vi "平均取樣數值適應性控制.vi"() -> ()   [LabVIEW 2010]
panel:
  in  "number of samples":i32=100
  in  "rate":dbl=1000.0
  in  "連續取樣多少誤差個數符合條件時算收斂":dbl=10.0
  in  "負誤差範圍%":dbl=-10.0
  in  "正誤差範圍%":dbl=10.0
  out "理想系統與FIR輸出":cluster{dbl, dbl}(graph)
  out "收斂時間":dbl
  out "Boolean":bool
  out "當下符合誤差條件數":dbl
  out "每次迴圈運時時間(ms)":u32
  out "當下誤差%":dbl
  out "error out":errorcluster
  out "system輸出":dbl
  out "input_x(t)":dbl(graph)
  out "ERR":dbl(graph)
  out "權重函數向量":dbl[](array[numeric])
  in  "order":i32=8
  out "LMS":dbl[](graph)
  out "FIR輸出":dbl
  in  "Stop Button":bool
  in  "u(收斂係數)":dbl=0.005
  # "A0:模擬輸入 pulse_output 2"
  # "A1:理想系統 pulse_output 1"
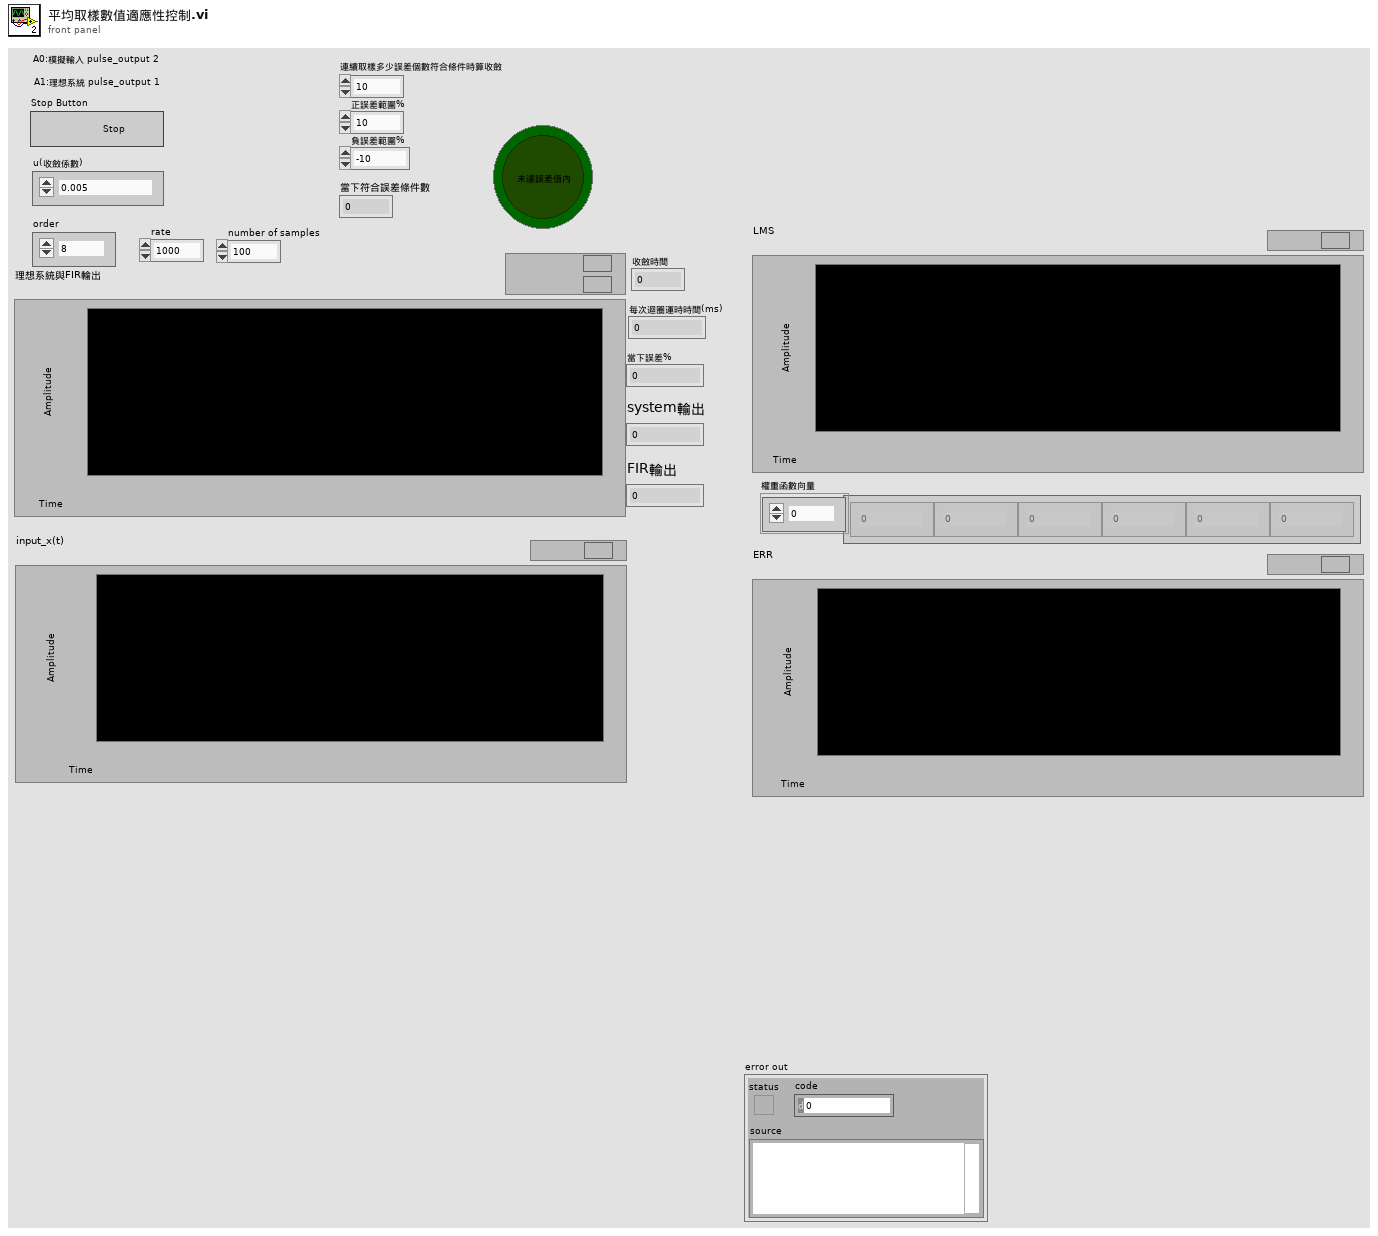
[diagram p1: front panel]
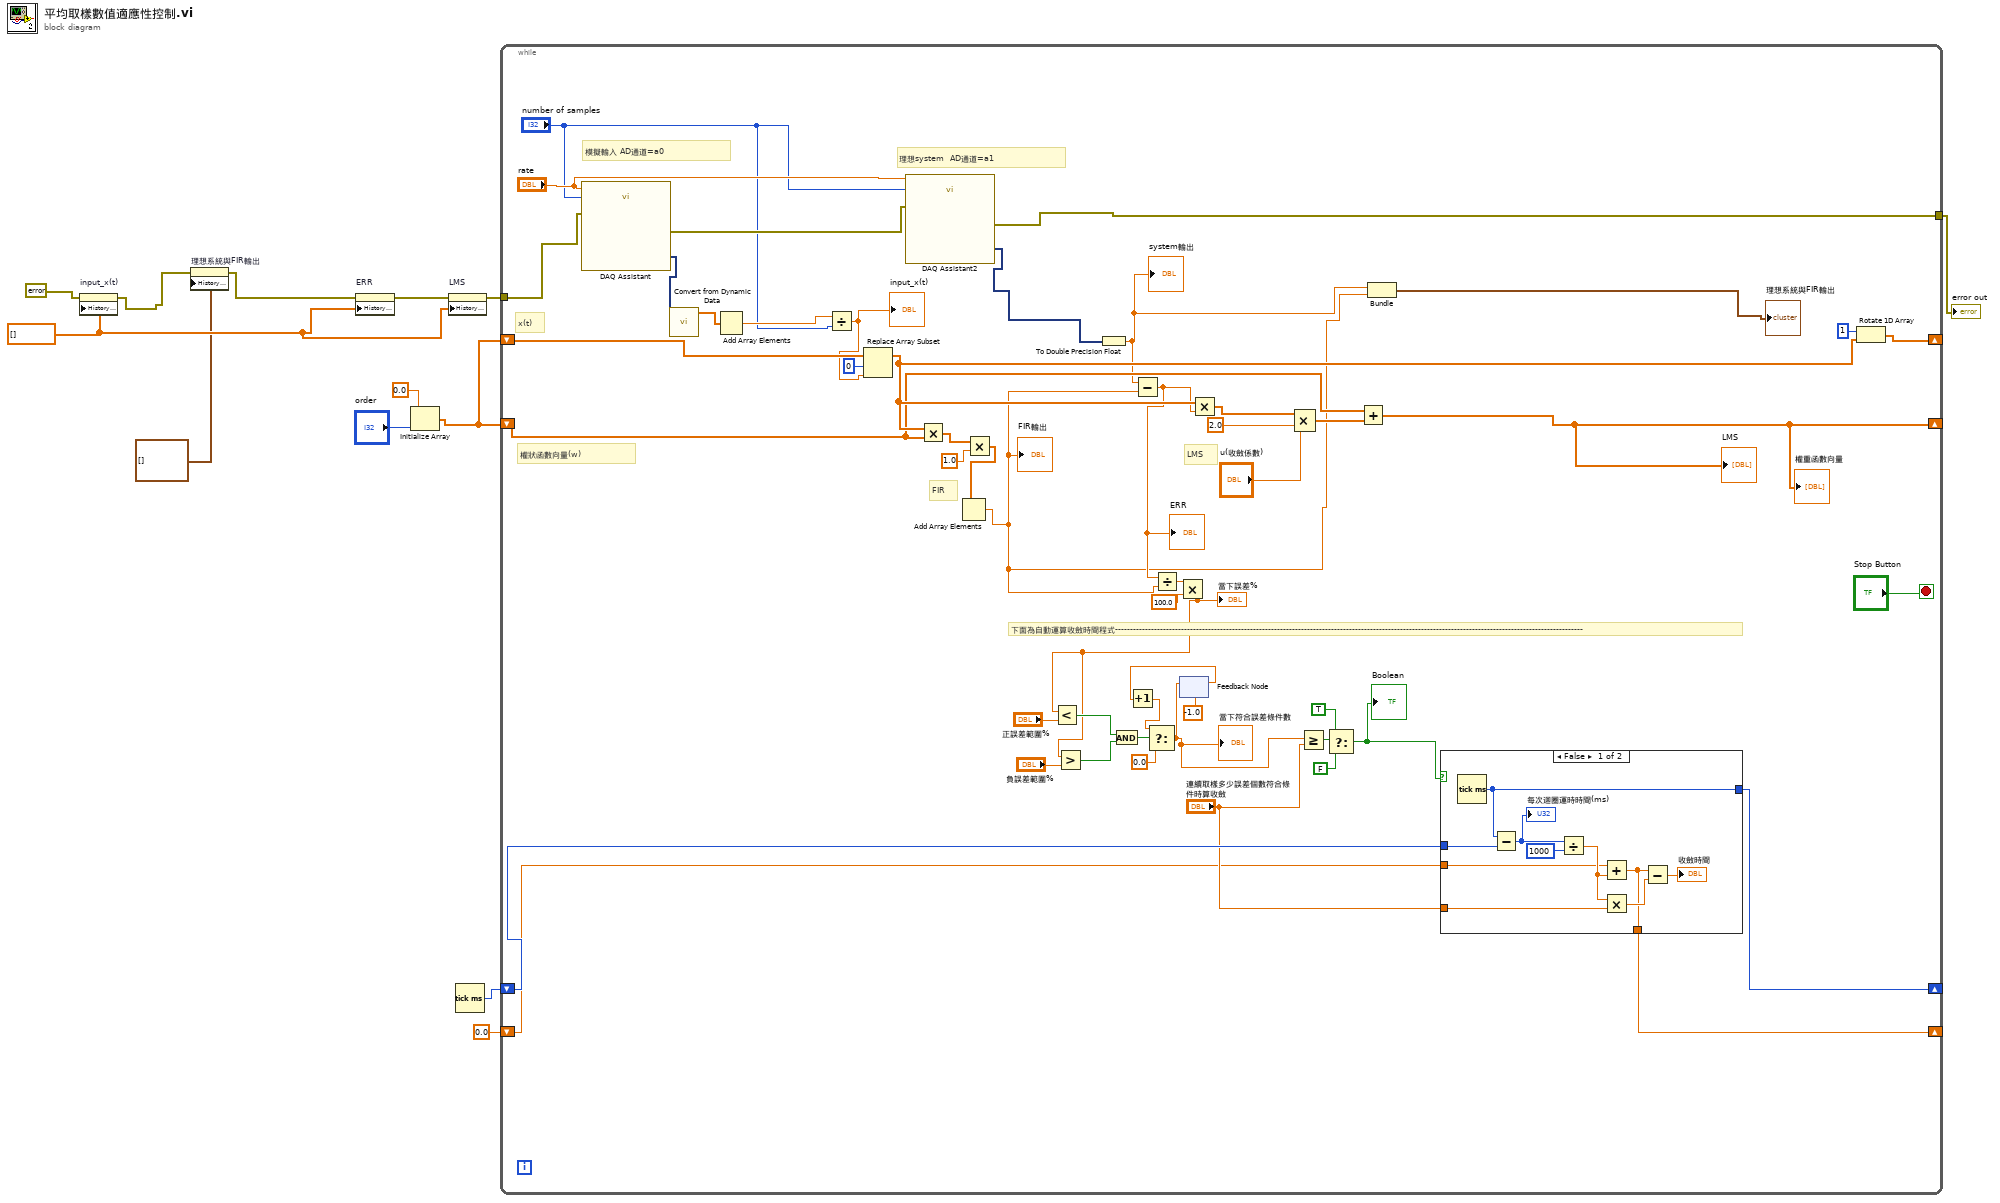
[diagram p0: block diagram]
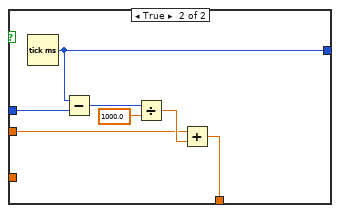
[diagram p2: hidden frame]
diagram:
  w9 = dbl[] [] ("History Data")
  n1 = property on="input_x(t)" class="WFChart (strict)"(error in=errorcluster {"status"=FALSE, "code"=0, "source"=""} ("error constant"), "History Data"=w9) -> (error out=w3:errorcluster)  [unwired: 1 in, 1 out]
  n2 = property on="理想系統與FIR輸出" class="WFChart (strict)"(error in=w3, "History Data"=cluster{dbl, dbl}[] []) -> (error out=w2:errorcluster)  [unwired: 1 in, 1 out]
  n3 = property on="ERR" class="WFChart (strict)"(error in=w2, "History Data"=w9) -> (error out=w7:errorcluster)  [unwired: 1 in, 1 out]
  n4 = Initialize Array "Initialize Array"(0.0 ("element"), "order") -> (w11:dbl[])
  n5 = property on="LMS" class="WFChart (strict)"(error in=w7, "History Data"=w9) -> (error out=w8:errorcluster)  [unwired: 1 in, 1 out]
  n6 = Tick Count (ms)() -> (millisecond timer value=w6:u32)
  n7 = while {
    shift-right: [w55] -> _
    shift-left: w11 -> [w54]
    shift-right: [w51] -> _
    shift-left: w11 -> [w50]
    tunnel: w8 -> [w45]
    shift-right: [w24] -> _
    shift-left: w6 -> [w25]
    shift-right: [w21] -> _
    shift-left: 0.0 ("index") -> [w22]
    tunnel: [w43] -> w4
    stop <- "Stop Button" stop-if-true
    # "下面為自動運算收斂時間程式------------------------------------------------------------------------------------------------------------------------------------------------------------"
    # "LMS"
    # "FIR"
    # "模擬輸入 AD通道=a0"
    # "權狀函數向量(w)"
    # "x(t)"
    # "理想system  AD通道=a1"
    n8 = call "DAQ Assistant"("rate"="rate", "number of samples"="number of samples", "error in"=w45) -> ("data"=w18:dynamicdata, "error out"=w44:errorcluster)  [unwired: 14 in, 1 out]
    n9 = call "Convert from Dynamic Data"("Dynamic Data Type"=w18) -> ("Array"=w17:dbl[])  [unwired: 3 in]
    n10 = Add Array Elements(numeric array=w17) -> (sum=w19:dbl)
    n11 = Divide(x=w19, y="number of samples") -> (x/y=w16:dbl)
    "input_x(t)" <- w16
    n12 = Replace Array Subset "Replace Array Subset"(array=w54, new element=w16, index=0) -> (w52:dbl[])
    n13 = call "DAQ Assistant2"("rate"="rate", "number of samples"="number of samples", "error in"=w44) -> ("data"=w46:dynamicdata, "error out"=w43:errorcluster)  [unwired: 14 in, 1 out]
    n14 = Multiply(x=w52, y=w50) -> (x*y=w64:dbl[])
    n15 = Multiply(x=w64, y=1.0) -> (x*y=w57:dbl[])
    n16 = Add Array Elements(numeric array=w57) -> (sum=w20:dbl)
    "FIR輸出" <- w20
    n17 = To Double Precision Float(number=w46) -> (double precision float=w29:dbl)
    "system輸出" <- w29
    n18 = Subtract(x=w29, y=w20) -> (x-y=w49:dbl)
    "ERR" <- w49
    n19 = Divide(x=w49, y=w20) -> (x/y=w48:dbl)
    n20 = Multiply(x=w48, y=100.0) -> (x*y=w32:dbl)
    "當下誤差%" <- w32
    n21 = Less?(x=w32, y="正誤差範圍%") -> (x < y?=w42:bool)
    n22 = Greater?(x=w32, y="負誤差範圍%") -> (0:w41:bool)
    n23 = And(x=w42, y=w41) -> (x .and. y?=w40:bool)
    n24 = feedback #1(-1.0) -> (w31:dbl)
    n25 = Increment(x=w31) -> (x+1=w38:dbl)
    n26 = Select(t=w38, s=w40, f=0.0) -> (s? t:f=w33:dbl)
    "當下符合誤差條件數" <- w33
    n27 = feedback-in #1(w33) -> ()
    n28 = Multiply(x=w52, y=w49) -> (x*y=w62:dbl[])
    n29 = Compound Arithmetic op=MULTIPLY(w62, 2.0 ("value"), "u(收斂係數)") -> (w59:dbl[])
    n30 = Greater Or Equal?(x=w33, y="連續取樣多少誤差個數符合條件時算收斂") -> (x >= y?=w36:bool)
    n31 = Select(t=TRUE, s=w36, f=FALSE) -> (s? t:f=w30:bool)
    "Boolean" <- w30
    n32 = Add(x=w50, y=w59) -> (x+y=w51:dbl[])
    "LMS" <- w51
    "權重函數向量" <- w51
    n33 = Bundle(w29, w20) -> (→"理想系統與FIR輸出":cluster{dbl, dbl})  [unwired: 1 in]
    n34 = case shown="False" w30 {
      tunnel: w25 -> [w73 w81]
      tunnel: [w72 w80] -> w24
      tunnel: "連續取樣多少誤差個數符合條件時算收斂" -> [w69 _]
      tunnel: w22 -> [w66 w76]
      tunnel: [w65 w75] -> w21
      frame False {
        n35 = Tick Count (ms)() -> (millisecond timer value=w72:u32)
        n36 = Subtract(x=w72, y=w73) -> (x-y=w70:u32)
        "每次迴圈運時時間(ms)" <- w70
        n37 = Divide(x=w70, y=u32 1000) -> (x/y=w67:dbl)
        n38 = Add(x=w66, y=w67) -> (x+y=w65:dbl)
        n39 = Multiply(x=w67, y=w69) -> (x*y=w68:dbl)
        n40 = Subtract(x=w65, y=w68) -> (x-y=→"收斂時間":dbl)
      }
      frame True {
        n41 = Tick Count (ms)() -> (millisecond timer value=w80:u32)
        n42 = Subtract(x=w80, y=w81) -> (x-y=w78:u32)
        n43 = Divide(x=w78, y=1000.0) -> (x/y=w77:dbl)
        n44 = Add(x=w76, y=w77) -> (x+y=w75:dbl)
      }
    }
    n45 = Rotate 1D Array(1:w52, 2:1 ("n")) -> (0:w55:dbl[])
  }
  "error out" <- w4
